vi "set_cameraName.vi"(0 "HGF_IMAQDevice":refnum<class "HGF_IMAQDevice.lvclass">, 2 "cameraName":string, 5 "error in (no error)":errorcluster) -> (14 "dup HGF_IMAQDevice":refnum<class "HGF_IMAQDevice.lvclass">, 19 "error out":errorcluster)   [LabVIEW 2014, in "HGF_IMAQ.lvlib" / "HGF_IMAQDevice.lvclass"]
doc: "Set name of camera."
uses:
  HGF_IMAQDevice.lvclass
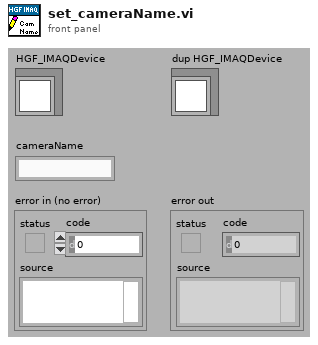
[diagram p1: front panel]
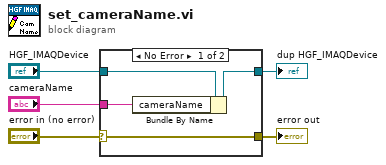
[diagram p0: block diagram]
diagram:
  n1 = case shown="No Error" "error in (no error)" {
    selector: "error in (no error)" -> [w9 w10]
    tunnel: [w9 w10] -> w4
    tunnel: [w7 w11] -> w2
    tunnel: "HGF_IMAQDevice" -> [w8 w11]
    tunnel: "cameraName" -> [w6 _]
    frame No Error {
      n2 = Bundle By Name(cluster=w8, "cameraName"=w6) -> (w7:refnum<class "HGF_IMAQDevice.lvclass">)
    }
    frame Error {
    }
  }
  "error out" <- w4
  "dup HGF_IMAQDevice" <- w2
